vi "getDescription.vi"(8 "error in (no error)":errorcluster, 11 "Espresso in":refnum<class "Espresso.lvclass">) -> (0 "error out":errorcluster, 2 "description":string, 3 "Espresso out":refnum<class "Espresso.lvclass">)   [LabVIEW 2013, in "Espresso.lvclass"]
uses:
  Espresso.lvclass
  Beverage/Beverage.lvclass
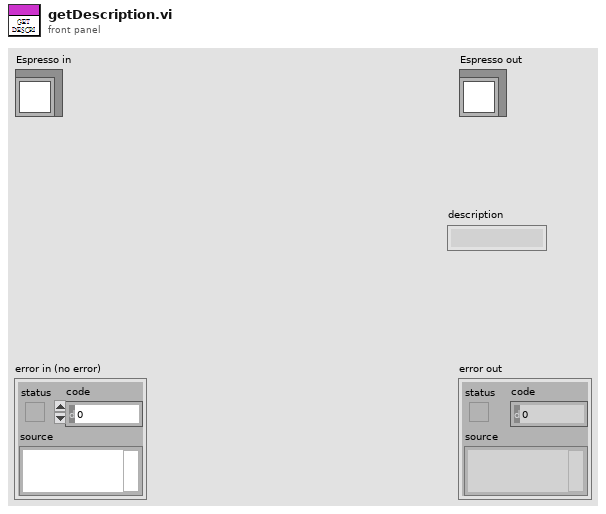
[diagram p1: front panel]
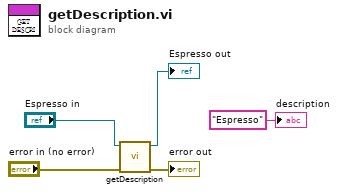
[diagram p0: block diagram]
diagram:
  n1 = call-parent "getDescription.vi"("error in (no error)"="error in (no error)", "Beverage in"="Espresso in") -> ("error out"=→"error out":errorcluster, "Beverage out"=→"Espresso out":refnum<class "Espresso.lvclass">)  [unwired: 7 in, 1 out]
  "description" <- "Espresso" ("description")
